vi "auto time.vi"() -> ()   [LabVIEW 2016]
panel:
  out "4U70 71M3":dbl
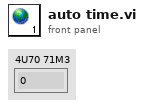
[diagram p1: front panel]
diagram:
